vi "control.vi"(5 "control":T5={"time (global)"=0.0, "MPV"=0, "manual control"={"sequence manual"=enum."WAIT", "sequence manual ?"=FALSE}}, 7 "command parameter":T1={"CO2 ref"=392.0, "CO2 span"=372.0, "H2O ref"=0.0, "H2O span"=0.0, "Zi"=0.0, "Zt"=1.2, "Zm"=0.0, "S"=0.0, "Temp [C]"=50.0, "Pressure [hPa]"=135.0, "Licor-Sources"=["CO2A W", "CO2B W", "H2OA W", "H2OB W", "T C", "T V", "P kPa", "P V", "RH %", "CO2A um/m", "CO2B um/m", "H2OA mm/m", "H2OB mm/m"], "Licor-Pump"="Off", "Zeitstempel"=timestamp(0 s since 1904-01-01)} {"Pressure [hPa]" format="%.2g"; "Temp [C]" format="%.2f"; "CO2 ref" format="%.2f"; "CO2 span" format="%.2g"; "H2O ref" format="%.2g"; "H2O span" format="%.2g"}, 8 "Licor-output":string[](array[string]), 9 "sequence in":T6={"sequence"=enum."WAIT", "time (next command)"=0.0}, 11 "command queue in":cluster{"Zeit [s]":i32, "Befehl":string}[](array[cluster])) -> (0 "Licor command":string, 1 "sequence out":T6={"sequence"=enum."WAIT", "time (next command)"=0.0}, 3 "command queue out":cluster{"Zeit [s]":i32, "Befehl":string}[](array[cluster]), 4 "data":string[](array[string]))   [LabVIEW 2010]
uses:
  Licor-Sequences.ctl
  Licor-Parameter.ctl
  Licor-Steuerung/LicorLI7000/conventions/Licor-Source.ctl
  Licor-Pump.ctl
  Licor-Steuerung/LicorLI7000/LicorLI7000.lvlib
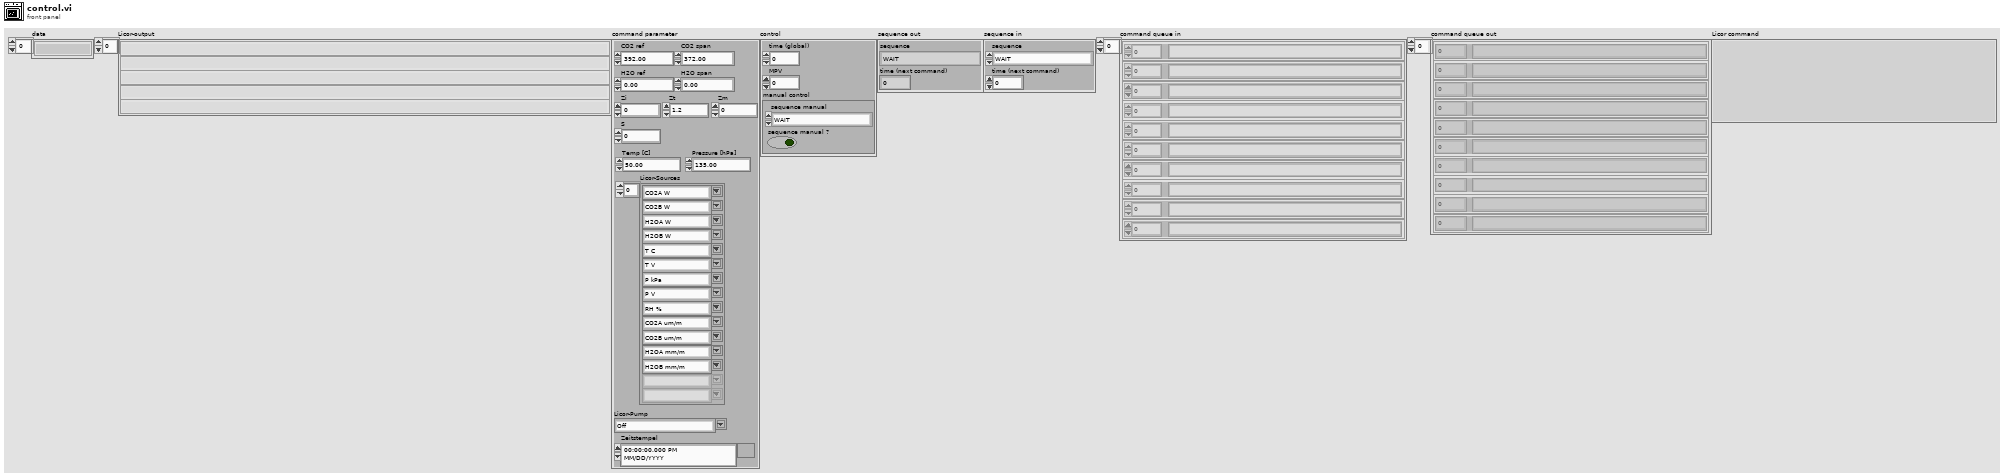
[diagram p1: front panel]
types:
  T1 = typedef "Licor-Parameter.ctl" = cluster{"CO2 ref":dbl, "CO2 span":dbl, "H2O ref":dbl, "H2O span":dbl, "Zi":dbl, "Zt":dbl, "Zm":dbl, "S":dbl, "Temp [C]":dbl, "Pressure [hPa]":dbl, "Licor-Sources":T2[], "Licor-Pump":T3, "Zeitstempel":timestamp}
  T2 = typedef "LicorLI7000.lvlib/Licor-Source.ctl" = string
  T3 = typedef "Licor-Pump.ctl" = string
  T4 = typedef "Licor-Sequences.ctl" = enum16{"test", "WAIT", "warmup", "initialize", "calibrate Z", "calibrate S"}
  T5 = cluster{"time (global)":dbl, "MPV":i32, "manual control":cluster{"sequence manual":T4, "sequence manual ?":bool}}
  T6 = cluster{"sequence":T4, "time (next command)":dbl}
  T7 = cluster{"sequence manual":T4, "time (next command)":dbl}
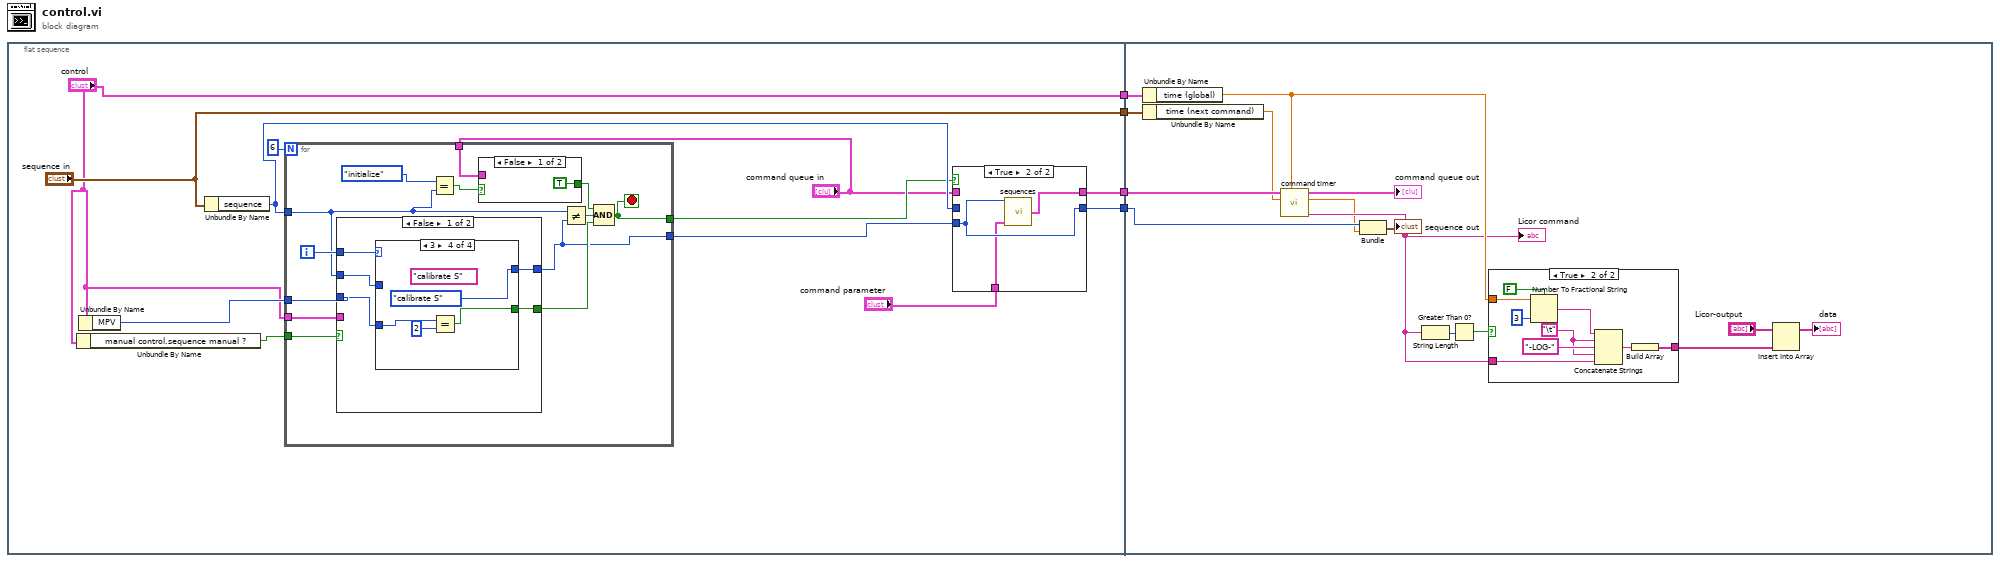
[diagram p0: block diagram]
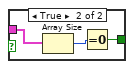
[diagram p3: hidden frame]
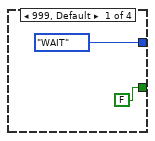
[diagram p4: hidden frame]
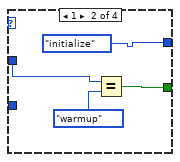
[diagram p5: hidden frame]
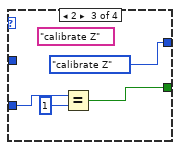
[diagram p6: hidden frame]
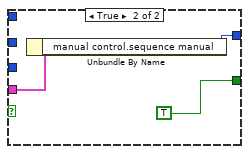
[diagram p7: hidden frame]
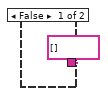
[diagram p8: hidden frame]
diagram:
  n1 = flat-sequence {
    tunnel: [w13] -> w4
    tunnel: [w11] -> w3
    tunnel: ["control"] -> w2
    tunnel: ["sequence in"] -> w1
    tunnel: w1 -> [w69]
    tunnel: w2 -> [w70]
    tunnel: w3 -> [w64]
    tunnel: w4 -> [w72]
    frame #0 {
      n2 = Unbundle By Name("control") -> ("manual control.sequence manual ?"=w14:bool)
      n3 = Unbundle By Name("control") -> ("MPV"=w15:i32)
      n4 = Unbundle By Name("sequence in") -> ("sequence"=w12:T4)
      n5 = for {
        N: 6 -> [_]
        tunnel: w15 -> [w33]
        tunnel: w12 -> [w22]
        tunnel: w14 -> [w30]
        tunnel: "control" -> [w29]
        tunnel: [w24] -> w10
        tunnel: [w28] -> w9
        tunnel: "command queue in" -> [w27]
        i -> [w34]
        stop <- w28 stop-if-true
        n6 = case shown="False" w30 {
          tunnel: w34 -> [w43 _]
          tunnel: w33 -> [w42 _]
          tunnel: [w41 w59] -> w24
          tunnel: [w40 TRUE] -> w31
          tunnel: w22 -> [w39 _]
          tunnel: w29 -> [_ w60]
          frame False {
            n7 = case shown="3" w43 {
              tunnel: w42 -> [_ _ w53 w56]
              tunnel: [FALSE w48 w51 w55] -> w40
              tunnel: [Licor-Sequences."WAIT" Licor-Sequences."initialize" Licor-Sequences."calibrate Z" Licor-Sequences."calibrate S"] -> w41
              tunnel: w39 -> [_ w49 _ _]
              frame 999, Default {
              }
              frame 1 {
                n8 = Equal?(x=w49, y=Licor-Sequences."warmup") -> (x = y?=w48:bool)
              }
              frame 2 {
                (unwired) "calibrate Z" ("sequence")
                n9 = Equal?(x=w53, y=1) -> (x = y?=w51:bool)
              }
              frame 3 {
                (unwired) "calibrate S" ("sequence")
                n10 = Equal?(x=w56, y=2) -> (x = y?=w55:bool)
              }
            }
          }
          frame True {
            n11 = Unbundle By Name(w60) -> ("manual control.sequence manual"=w59:T4)
          }
        }
        n12 = Equal?(x=Licor-Sequences."initialize", y=w22) -> (x = y?=w26:bool)
        n13 = case shown="False" w26 {
          tunnel: w27 -> [_ w37]
          tunnel: [TRUE w36] -> w25
          frame False {
          }
          frame True {
            n14 = Array Size(array=w37) -> (size(s)=w38:i32)
            n15 = Equal To 0?(x=w38) -> (x = 0?=w36:bool)
          }
        }
        n16 = Not Equal?(x=w22, y=w24) -> (x != y?=w32:bool)
        n17 = Compound Arithmetic op=AND(w25, w32, w31) -> (w28:bool)
      }
      n18 = case shown="True" w9 {
        tunnel: "command queue in" -> [w18 _]
        tunnel: [w18 w21] -> w13
        tunnel: w12 -> [w17 _]
        tunnel: [w17 w20] -> w11
        tunnel: w10 -> [_ w20]
        tunnel: "command parameter" -> [_ w19]
        frame False {
        }
        frame True {
          n19 = call "sequences.vi"("sequence"=w20, "command parameter"=w19) -> ("sequence out"=w21:cluster{"time":i32, "command":string}[])  [unwired: 13 in]
        }
      }
    }
    frame #1 {
      n20 = Unbundle By Name(w70) -> ("time (global)"=w68:dbl)
      n21 = Unbundle By Name(w69) -> ("time (next command)"=w63:dbl)
      n22 = call "command timer.vi"("time (global)"=w68, "time (next command)"=w63, "command queue in"=w72) -> ("Licor command"=w65:string, "time (next command)"=w61:dbl, "command queue out"=→"command queue out":cluster{"Zeit [s]":i32, "Befehl":string}[])  [unwired: 6 in]
      "Licor command" <- w65
      n23 = Bundle("sequence manual"=w64, "time (next command)"=w61) -> (→"sequence out":T7)  [unwired: 1 in]
      n24 = String Length(string=w65) -> (length=w67:i32)
      n25 = Greater Than 0?(x=w67) -> (x > 0?=w66:bool)
      n26 = case shown="True" w66 {
        tunnel: w68 -> [_ w85]
        tunnel: w65 -> [_ w81]
        tunnel: [string[] [] w79] -> w74
        frame False {
        }
        frame True {
          w82 = "\t"
          n27 = Number To Fractional String(use system decimal point (T)=FALSE ("Systemdezimalzeichen verwenden (T)"), number=w85, precision (6)=i16 3 ("Genauigkeit (6)")) -> (F-format string=w84:string)  [unwired: 1 in]
          n28 = Concatenate Strings(w84, w82, "-LOG-", w82, w81) -> (w80:string)
          n29 = Build Array(w80) -> (w79:string[])
        }
      }
      n30 = Insert Into Array(array="Licor-output", new element=w74) -> (→"data":string[])  [unwired: 1 in]
    }
  }
